vi "Autonomous Rotation.vi"(9 "PID gains":T1={"proportional gain (Kc)"=0.025, "integral time (Ti, min)"=0.0, "derivative time (Td, min)"=0.001} {"derivative time (Td, min)" format="%.3f"; "integral time (Ti, min)" format="%.3f"; "proportional gain (Kc)" format="%.3f"}, 10 "Rotation Speed":dbl format="%#_13g", 11 "Desired Angle":dbl format="%#_13g") -> ()   [LabVIEW 2014]
uses:
  Controls/SRE Enum.ctl
  Support Code/Robot Global Data.vi
  <vilib>/addons/control/pid/pid.llb/PID (DBL).vi
  <vilib>/addons/control/pid/NI_PID_pid.lvlib
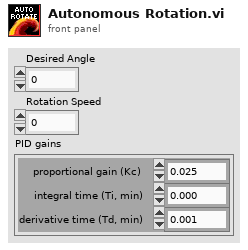
[diagram p1: front panel]
types:
  T1 = cluster{"proportional gain (Kc)":dbl, "integral time (Ti, min)":dbl, "derivative time (Td, min)":dbl}
  T2 = typedef "SRE Enum.ctl" = enum16{"Start", "Run", "End"}
  T3 = cluster{"Speed":dbl, "Direction":dbl, "Rotation":dbl}
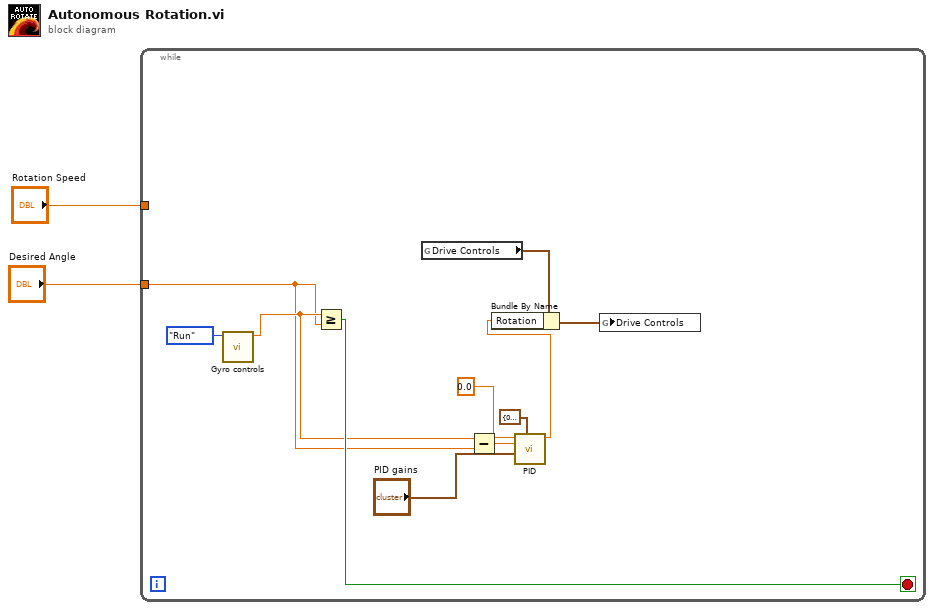
[diagram p0: block diagram]
diagram:
  n1 = while {
    tunnel: "Desired Angle" -> [w6]
    tunnel: "Rotation Speed" -> [_]
    stop <- w10 stop-if-true
    n2 = call "Gyro controls.vi"("Enum"=SRE_Enum."Run") -> ("Angle"=w7:dbl)  [unwired: 10 in]
    n3 = Greater Or Equal?(x=w7, y=w6) -> (x >= y?=w10:bool)
    n4 = global read "Robot Global Data.vi" "Drive Controls"() -> (w12:T3)
    n5 = Subtract(x=w7, y=w6) -> (x-y=w8:dbl)
    n6 = call-poly <vilib>:"PID.vi"("output range"=cluster{"output high":dbl, "output low":dbl} {"output high"=0.5, "output low"=-0.5}, "PID gains"="PID gains", "process variable"=w8, "setpoint"=0.0) -> ("output"=w4:dbl)  [unwired: 6 in, 1 out]
    n7 = Bundle By Name(cluster=w12, "Rotation"=w4) -> (w11:T3)
    n8 = global write "Robot Global Data.vi" "Drive Controls"(w11) -> ()
  }
